vi "DRIVE_POWER.vi"(10 "argv":string[](array[string]), 11 "args":u8) -> ()   [LabVIEW 2011]
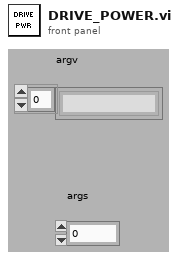
[diagram p1: front panel]
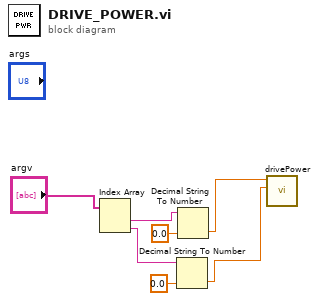
[diagram p0: block diagram]
diagram:
  n1 = Index Array(array="argv") -> (element #1=w6:string, element #2=w2:string)  [unwired: 2 in]
  n2 = Decimal String To Number(string=w2, default (0L)=0.0 ("default (0 I32)")) -> (number=w1:dbl)  [unwired: 1 in, 1 out]
  n3 = Decimal String To Number(string=w6, default (0L)=0.0 ("default (0 I32)")) -> (number=w5:dbl)  [unwired: 1 in, 1 out]
  n4 = call "drivePower.vi"("speed"=w1, "time"=w5) -> ()  [unwired: 10 in]
